vi "aggState.vi"(8 "error in (no error)":errorcluster, 10 "State in DOF":dbl[](array[numeric]), 11 "ZTAAC in":refnum<class "ZTAAC.lvclass">) -> (0 "error out":errorcluster, 3 "ZTAAC out":refnum<class "ZTAAC.lvclass">)   [LabVIEW 2016, in "OfcFunc.lvlib" / "ZTAAC.lvclass"]
doc: "Aggregate the calculated degree of freedom (DOF) in the state."
uses:
  ZTAAC.lvclass
  ZTAAC.lvclass/ZTAAC.ctl
  OptStateEsti/OptStateEsti.lvclass
  OptCtrl/OptCtrl.lvclass
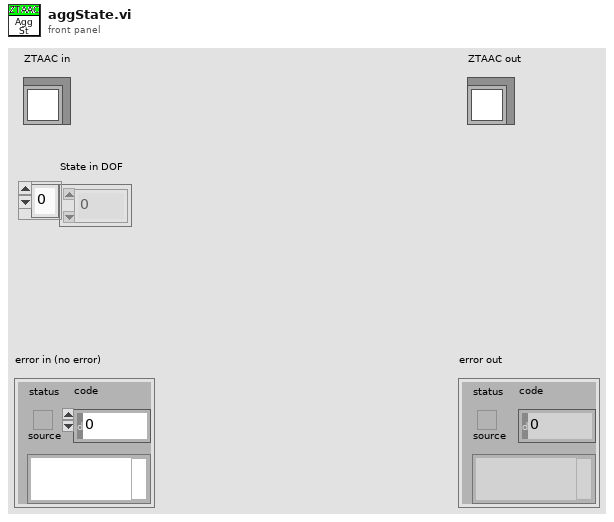
[diagram p1: front panel]
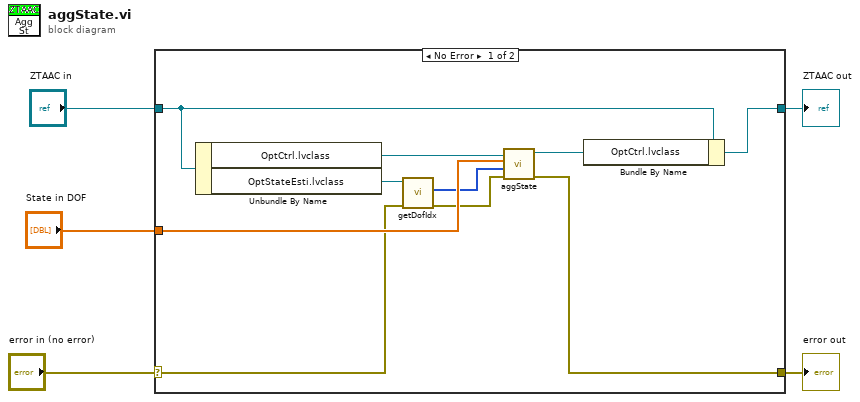
[diagram p0: block diagram]
diagram:
  n1 = case shown="No Error" "error in (no error)" {
    selector: "error in (no error)" -> [w8 w17]
    tunnel: [w6 w17] -> w4
    tunnel: [w9 w16] -> w2
    tunnel: "ZTAAC in" -> [w11 w16]
    tunnel: "State in DOF" -> [w13 _]
    frame No Error {
      n2 = Unbundle By Name(w11) -> ("OptCtrl.lvclass"=w14:refnum<class "OptCtrl.lvclass">, "OptStateEsti.lvclass"=w15:refnum<class "OptStateEsti.lvclass">)
      n3 = call "getDofIdx.vi"("error in (no error)"=w8, "OptStateEsti in"=w15) -> ("error out"=w7:errorcluster, "dofIdx"=w12:i32[])  [unwired: 7 in, 1 out]
      n4 = call "aggState.vi"("error in (no error)"=w7, "dofIdx"=w12, "State in DOF"=w13, "OptCtrl in"=w14) -> ("error out"=w6:errorcluster, "OptCtrl out"=w10:refnum<class "OptCtrl.lvclass">)  [unwired: 6 in]
      n5 = Bundle By Name(cluster=w11, "OptCtrl.lvclass"=w10) -> (w9:refnum<class "ZTAAC.lvclass">)
    }
    frame Error {
    }
  }
  "error out" <- w4
  "ZTAAC out" <- w2
